vi "LVClass_HasoData Get Compute Slopes Set - StartPupils Size.vi"(0 "HasoData in":refnum<class "HasoData.lvclass">, 11 "error in (no error)":errorcluster) -> (4 "HasoData out":refnum<class "HasoData.lvclass">, 8 "Size":i32 min=0 max=1, 15 "error out":errorcluster)   [LabVIEW 2020, in "HasoData.lvclass"]
doc: "HasoSlopes computation preferences getter.\n\n--------------------------------------------------------------------------------\n\n<B>HasoEngineIn </B> : HasoEngine object.\n<B>HasoEngineOut </B> : HasoEngine object.\n<B>start_subpupil </B> : Coordinates of the first calculated sub-pupil (index coordinates relative to\n the top-left corner of the pupil).\n<B>denoising_strength </B> : Sensitivity of spot detection on summed images (between 0 and 1).\n<B>ErrorIn </B> : Error\n<B>ErrorOut </B> : Error\n\n--------------------------------------------------------------------------------"
uses:
  HasoData.lvclass
  HasoData.lvclass/HasoData.ctl
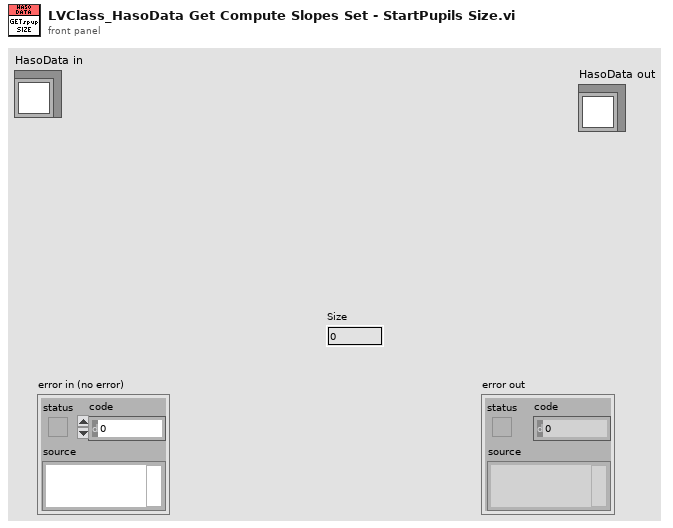
[diagram p1: front panel]
types:
  T1 = typedef "ClassID.ctl" = i64
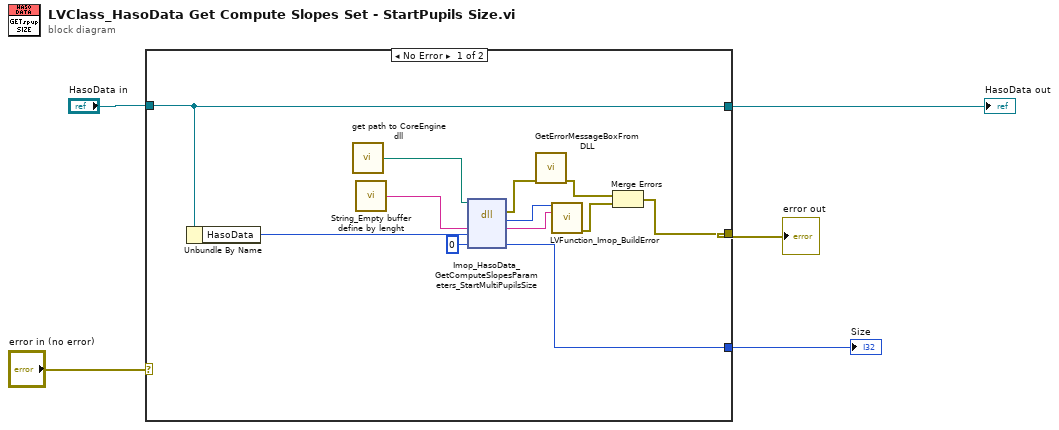
[diagram p0: block diagram]
diagram:
  n1 = case shown="No Error" "error in (no error)" {
    selector: "error in (no error)" -> [_ w18]
    tunnel: "HasoData in" -> [w12 w19]
    tunnel: [w12 w19] -> w1
    tunnel: [w8 w18] -> w4
    tunnel: [w7 _] -> w3
    frame No Error {
      n2 = Unbundle By Name(w12) -> ("HasoData"=w11:T1)
      n3 = call "get path to CoreEngine dll.vi"() -> ("path to wavekit library"=w14:path)  [unwired: 14 in, 1 out]
      n4 = call "String_Empty buffer define by lenght.vi"() -> ("Empty buffer"=w15:string)  [unwired: 1 in]
      n5 = dll-call lib="D:/2_trunk/Soft_haso/ImOpCoreEngine4_LV2011/DLLs/ImopEngine4_vc100.dll" fn="Imop_HasoData_GetComputeSlopesParameters_StartMultiPupilsSize"(path in=w14, "message"=w15, "objet"=w11, "pupil_average"=0) -> (error out=w13:errorcluster, "return type"=w16:i32, "message"=w17:string, "pupil_average"=w7:i32)  [unwired: 3 in, 1 out]
      n6 = call "GetErrorMessageBoxFromDLL.vi"("error IN"=w13) -> ("error OUT"=w10:errorcluster)  [unwired: 10 in]
      n7 = call "LVFunction_Imop_BuildError.vi"("code"=w16, "String to Prepend to source (\"\")"=w17) -> ("error out"=w9:errorcluster)  [unwired: 13 in]
      n8 = Merge Errors(w10, w9) -> (w8:errorcluster)
    }
    frame Error {
    }
  }
  "error out" <- w4
  "Size" <- w3
  "HasoData out" <- w1
